vi "calculate polarization.vi"(6 "background intensity":dbl, 8 "polarimeter angle":dbl, 9 "pressure factor":dbl, 10 "min":dbl, 11 "max":dbl) -> (3 "estimated polarization":dbl)   [LabVIEW 2018]
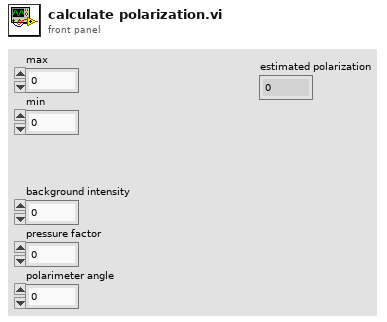
[diagram p1: front panel]
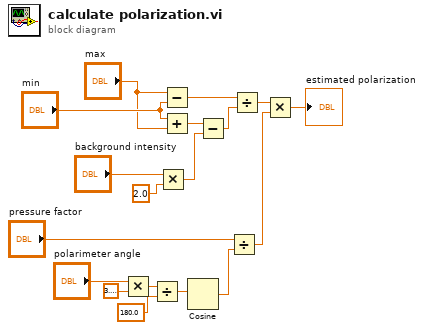
[diagram p0: block diagram]
diagram:
  n1 = Multiply(x="polarimeter angle", y=3.141592653589793) -> (x*y=w16:dbl)
  n2 = Divide(x=w16, y=180.0) -> (x/y=w14:dbl)
  n3 = Multiply(x="background intensity", y=2.0 ("x")) -> (x*y=w10:dbl)
  n4 = Subtract(x="max", y="min") -> (x-y=w6:dbl)
  n5 = Add(x="min", y="max") -> (x+y=w11:dbl)
  n6 = Cosine(x=w14) -> (cos(x)=w12:dbl)
  n7 = Subtract(x=w11, y=w10) -> (x-y=w9:dbl)
  n8 = Divide(x="pressure factor", y=w12) -> (x/y=w5:dbl)
  n9 = Divide(x=w6, y=w9) -> (x/y=w8:dbl)
  n10 = Multiply(x=w8, y=w5) -> (x*y=→"estimated polarization":dbl)
